vi "updateFilter.vi"(6 "Filter MED":T1, 8 "error in (no error)":errorcluster, 9 "AVG Filter type":T2, 10 "Filter":T1, 11 "ElectrometerController in":refnum<class "ElectrometerController.lvclass">) -> (0 "error out":errorcluster, 3 "ElectrometerController out":refnum<class "ElectrometerController.lvclass">)   [LabVIEW 2016, in "ElectrometerController.lvclass"]
uses:
  ElectrometerController.lvclass
  Electrometer/MED Filter Type.ctl
  Electrometer/AVG Filter type.ctl
  Electrometer/Electrometer.lvclass
  ElectrometerConfiguration/ElectrometerInternalConfiguration.lvclass
  Electrometer/State/ElectrometerState.lvclass
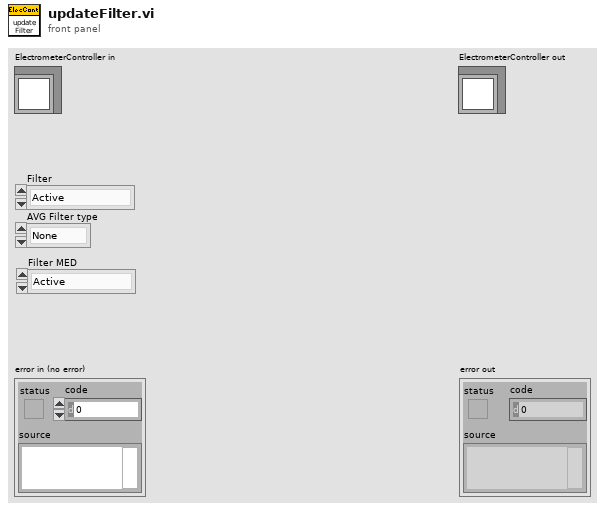
[diagram p1: front panel]
types:
  T1 = typedef "Electrometer.lvclass/MED Filter Type.ctl" = enum16{"Active", "None"}
  T2 = typedef "Electrometer.lvclass/AVG Filter type.ctl" = enum16{"None", "Scalar", "Advanced"}
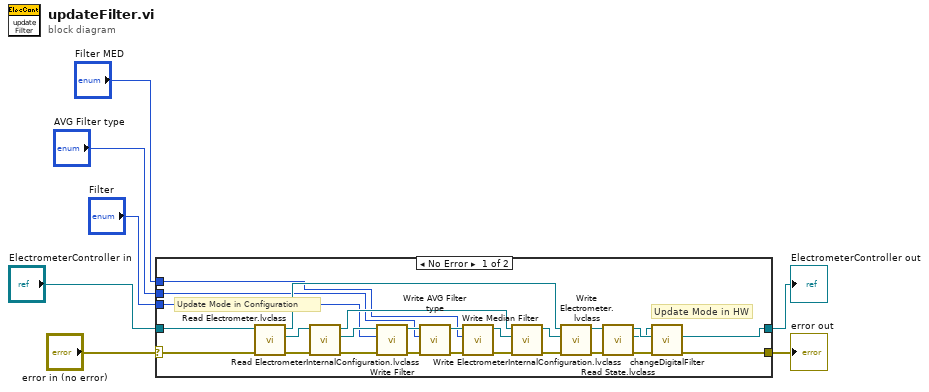
[diagram p0: block diagram]
diagram:
  n1 = case shown="No Error" "error in (no error)" {
    selector: "error in (no error)" -> [w17 w35]
    tunnel: [w15 w35] -> w6
    tunnel: [w14 w34] -> w4
    tunnel: "ElectrometerController in" -> [w16 w34]
    tunnel: "Filter" -> [w10 _]
    tunnel: "AVG Filter type" -> [w9 _]
    tunnel: "Filter MED" -> [w8 _]
    frame No Error {
      # "Update Mode in HW"
      # "Update Mode in Configuration"
      n2 = call-dynamic "Read Electrometer.lvclass.vi"("error in (no error)"=w17, "ElectrometerController in"=w16) -> ("error out"=w26:errorcluster, "Electrometer.lvclass"=w31:refnum<class "Electrometer.lvclass">, "ElectrometerController out"=w30:refnum<class "ElectrometerController.lvclass">)  [unwired: 7 in]
      n3 = call-dynamic "Read ElectrometerInternalConfiguration.lvclass.vi"("error in (no error)"=w26, "Electrometer in"=w31) -> ("error out"=w21:errorcluster, "ElectrometerInternalConfiguration.lvclass"=w22:refnum<class "ElectrometerInternalConfiguration.lvclass">, "Electrometer out"=w33:refnum<class "Electrometer.lvclass">)  [unwired: 7 in]
      n4 = call-dynamic "Write Filter.vi"("error in (no error)"=w21, "Filter"=w10, "ElectrometerInternalConfiguration in"=w22) -> ("error out"=w20:errorcluster, "ElectrometerInternalConfiguration out"=w23:refnum<class "ElectrometerInternalConfiguration.lvclass">)  [unwired: 7 in]
      n5 = call-dynamic "Write AVG Filter type.vi"("error in (no error)"=w20, "AVG Filter type"=w9, "ElectrometerInternalConfiguration in"=w23) -> ("error out"=w19:errorcluster, "ElectrometerInternalConfiguration out"=w24:refnum<class "ElectrometerInternalConfiguration.lvclass">)  [unwired: 7 in]
      n6 = call-dynamic "Write Median Filter.vi"("error in (no error)"=w19, "Filter"=w8, "ElectrometerInternalConfiguration in"=w24) -> ("error out"=w18:errorcluster, "ElectrometerInternalConfiguration out"=w25:refnum<class "ElectrometerInternalConfiguration.lvclass">)  [unwired: 7 in]
      n7 = call-dynamic "Write ElectrometerInternalConfiguration.lvclass.vi"("error in (no error)"=w18, "ElectrometerInternalConfiguration.lvclass"=w25, "Electrometer in"=w33) -> ("error out"=w29:errorcluster, "Electrometer out"=w32:refnum<class "Electrometer.lvclass">)  [unwired: 7 in]
      n8 = call-dynamic "Write Electrometer.lvclass.vi"("error in (no error)"=w29, "Electrometer.lvclass"=w32, "ElectrometerController in"=w30) -> ("error out"=w28:errorcluster, "ElectrometerController out"=w27:refnum<class "ElectrometerController.lvclass">)  [unwired: 7 in]
      n9 = call-dynamic "Read State.lvclass.vi"("error in (no error)"=w28, "ElectrometerController in"=w27) -> ("error out"=w13:errorcluster, "ElectrometerState"=w11:refnum<class "ElectrometerState.lvclass">, "ElectrometerController out"=w12:refnum<class "ElectrometerController.lvclass">)  [unwired: 7 in]
      n10 = call-dynamic "changeDigitalFilter.vi"("error in (no error)"=w13, "ElectrometerController in"=w12, "State in"=w11) -> ("error out"=w15:errorcluster, "ElectrometerController out"=w14:refnum<class "ElectrometerController.lvclass">)  [unwired: 6 in, 1 out]
    }
    frame Error {
    }
  }
  "error out" <- w6
  "ElectrometerController out" <- w4
